vi "ReDraw ROI - get Z planes.vi"() -> ()   [LabVIEW 2020]
panel:
  out "Z Motor INdex":i32[](array[numeric])
  in  "Motor Z":dbl[](array[numeric])
  in  "Z Stop":dbl
  in  "Z Start":dbl
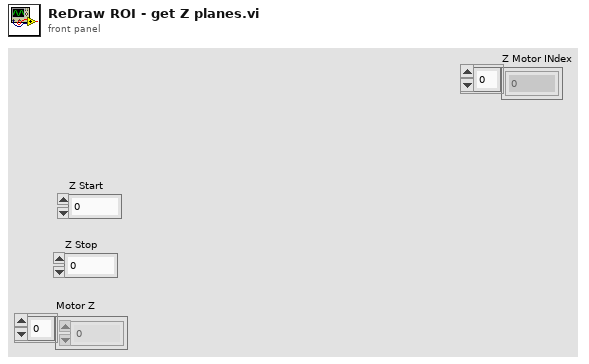
[diagram p1: front panel]
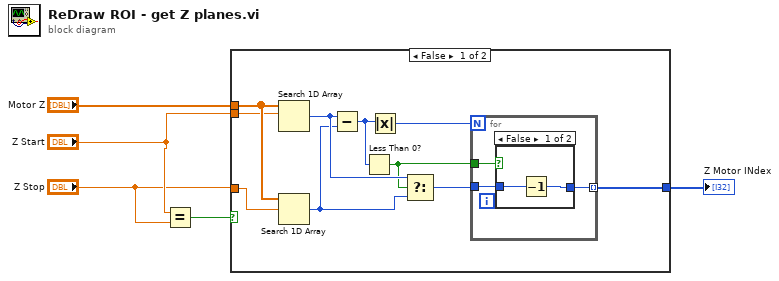
[diagram p0: block diagram]
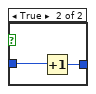
[diagram p2: hidden frame]
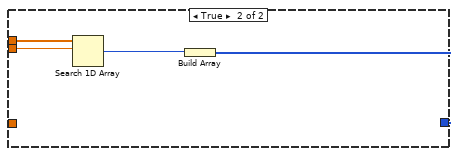
[diagram p3: hidden frame]
diagram:
  n1 = Equal?(x="Z Start", y="Z Stop") -> (x = y?=w2:bool)
  n2 = case shown="False" w2 {
    tunnel: "Motor Z" -> [w15 w26]
    tunnel: "Z Start" -> [w14 w25]
    tunnel: "Z Stop" -> [w13 _]
    tunnel: [w7 w23] -> w1
    frame False {
      n3 = Search 1D Array(1D array=w15, element=w14) -> (index of element=w10:i32)  [unwired: 1 in]
      n4 = Search 1D Array(1D array=w15, element=w13) -> (index of element=w9:i32)  [unwired: 1 in]
      n5 = Subtract(x=w10, y=w9) -> (x-y=w11:i32)
      n6 = Less Than 0?(x=w11) -> (x < 0?=w6:bool)
      n7 = Absolute Value(x=w11) -> (abs(x)=w12:i32)
      n8 = Select(t=w10, s=w6, f=w9) -> (s? t:f=w8:i32)
      n9 = for {
        N: w12 -> [_]
        tunnel: w8 -> [w18]
        tunnel: [w17] -> w7 mode=indexing
        tunnel: w6 -> [w16]
        n10 = case shown="False" w16 {
          tunnel: w18 -> [w19 w22]
          tunnel: [w20 w21] -> w17
          frame False {
            n11 = Decrement(x=w19) -> (x-1=w20:i32)
          }
          frame True {
            n12 = Increment(x=w22) -> (x+1=w21:i32)
          }
        }
      }
    }
    frame True {
      n13 = Search 1D Array(1D array=w26, element=w25) -> (index of element=w24:i32)  [unwired: 1 in]
      n14 = Build Array(w24) -> (w23:i32[])
    }
  }
  "Z Motor INdex" <- w1
